vi "Operation Main.vi"(8 "error in (no error)":errorcluster, 11 "Stand Alone Display Actor in":refnum<class "Stand Alone Display Actor.lvclass">) -> (0 "error out":errorcluster, 3 "Stand Alone Display Actor out":refnum<class "Stand Alone Display Actor.lvclass">)   [LabVIEW 2024, in "Stand Alone Display Actor.lvclass"]
uses:
  Stand Alone Display Actor.lvclass
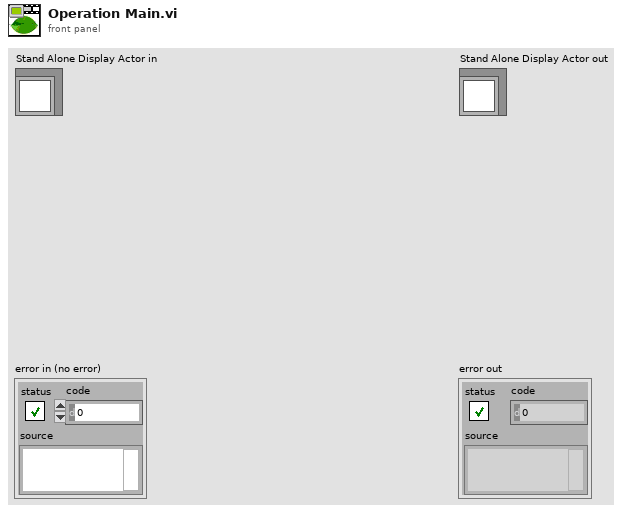
[diagram p1: front panel]
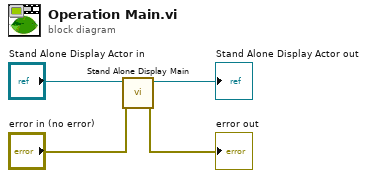
[diagram p0: block diagram]
diagram:
  n1 = call-dynamic "Stand Alone Display Main.vi"("error in (no error)"="error in (no error)", "Stand Alone Display Actor in"="Stand Alone Display Actor in") -> ("error out"=→"error out":errorcluster, "Stand Alone Display Actor out"=→"Stand Alone Display Actor out":refnum<class "Stand Alone Display Actor.lvclass">)  [unwired: 8 in]
